vi "logOCT.vi"(1 "vol":dbl[][][](array[numeric])) -> (0 "log vol":u16[][][](array[numeric]))   [LabVIEW 2017]
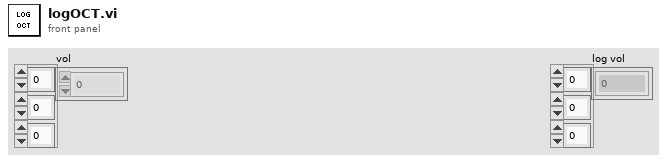
[diagram p1: front panel]
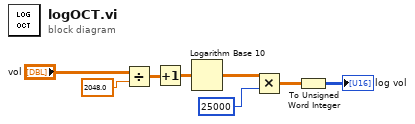
[diagram p0: block diagram]
diagram:
  n1 = Divide(x="vol", y=2048.0) -> (x/y=w7:dbl[][][])
  n2 = Increment(x=w7) -> (x+1=w6:dbl[][][])
  n3 = Logarithm Base 10(1:w6) -> (0:w5:dbl[][][])
  n4 = Multiply(x=w5, y=25000) -> (x*y=w3:dbl[][][])
  n5 = To Unsigned Word Integer(number=w3) -> (unsigned 16bit integer=→"log vol":u16[][][])
